vi "RT_FPGA_manualoffset_v8.vi"() -> ()   [LabVIEW 2015]
uses:
  <vilib>/rvi/interface/nirviReadWriteControl/nirviReadWriteControl.xnode
  <vilib>/rvi/interface/Simulation/niFpgaSimulationCallBeginRW.vi
  <vilib>/rvi/errors/niLvFpgaAdjustHostInterfaceError.vi
  <vilib>/rvi/interface/nirviOpenFPGA/nirviOpenFPGA.xnode
  NiFpgaLv.dll
  <vilib>/Utility/error.llb/Error Cluster From Error Code.vi
  FPGA_MPU_rev1.vi
panel:
  in  "delay in while loop execution (ms)":u32=10
  out "Acceleration (g)":cluster{dbl, dbl, dbl}(graph)
  out "Compass (deg)":cluster{dbl, dbl, dbl}(graph)
  out "Gyroscope(deg/s)":cluster{"x":dbl, "y":dbl, "z":dbl}(graph)
  in  "?":bool
  in  "stop data collection":bool
  in  "ZgyroOffH":dbl=5888.0 min=5888.0 max=6143.0
  in  "XgyroOffH":dbl=5119.0 min=4864.0 max=5119.0
  in  "YgyroOffH":dbl=5631.0 min=5376.0 max=5631.0
  in  "delay in while loop execution (ms)":u32=500
  in  "ZgyroOffL":dbl=6399.0 min=6144.0 max=6399.0
  in  "XgyroOffL":dbl=5350.0 min=5120.0 max=5375.0
  in  "YgyroOffL":dbl=5855.0 min=5632.0 max=5887.0
  in  "stop":bool
  in  "ZAccOffH":dbl=32034.0 min=32000.0 max=32255.0
  in  "XAccOffH":dbl=30483.0 min=30464.0 max=30719.0
  out "Array":u16[](array[numeric])=[5119, 5262, 5630, 5823, 5888, 6198, 6419, 6658, 6912, 7176, 7430, 7680, 7936, 8960, 14337, 14849, 27393, 30464, 30720, 31436, 31692, 32000, 32256, 27168, 26371, 6419, 6658, 14337, 14849, 9280, 9612, 9730, 10120, 10252, 10506, 10881, 25601, 27648]
  out "output array":u16[](array[numeric])
  in  "YAccOffH":dbl=31467.0 min=31232.0 max=31487.0
  out "Acceleration (g)":cluster{dbl, dbl, dbl}(graph)
  out "Gyroscope (deg/s)":cluster{dbl, dbl, dbl}(graph)
  out "Compass (deg)":cluster{dbl, dbl, dbl}(graph)
  out "array":u32[](array[numeric])
  # "Data collection"
  # "Offset"
  # "Offset control"
  # "30464 to 30719"
  # "31232 to 31487"
  # "32000 to 32255"
  # "Coarse"
  # "4864 to 5119"
  # "5376 to 5631"
  # "5888 to 6143"
  # "Fine"
  # "5120 to 5375"
  # "5632 to 5897"
  # "6144 to 6399"
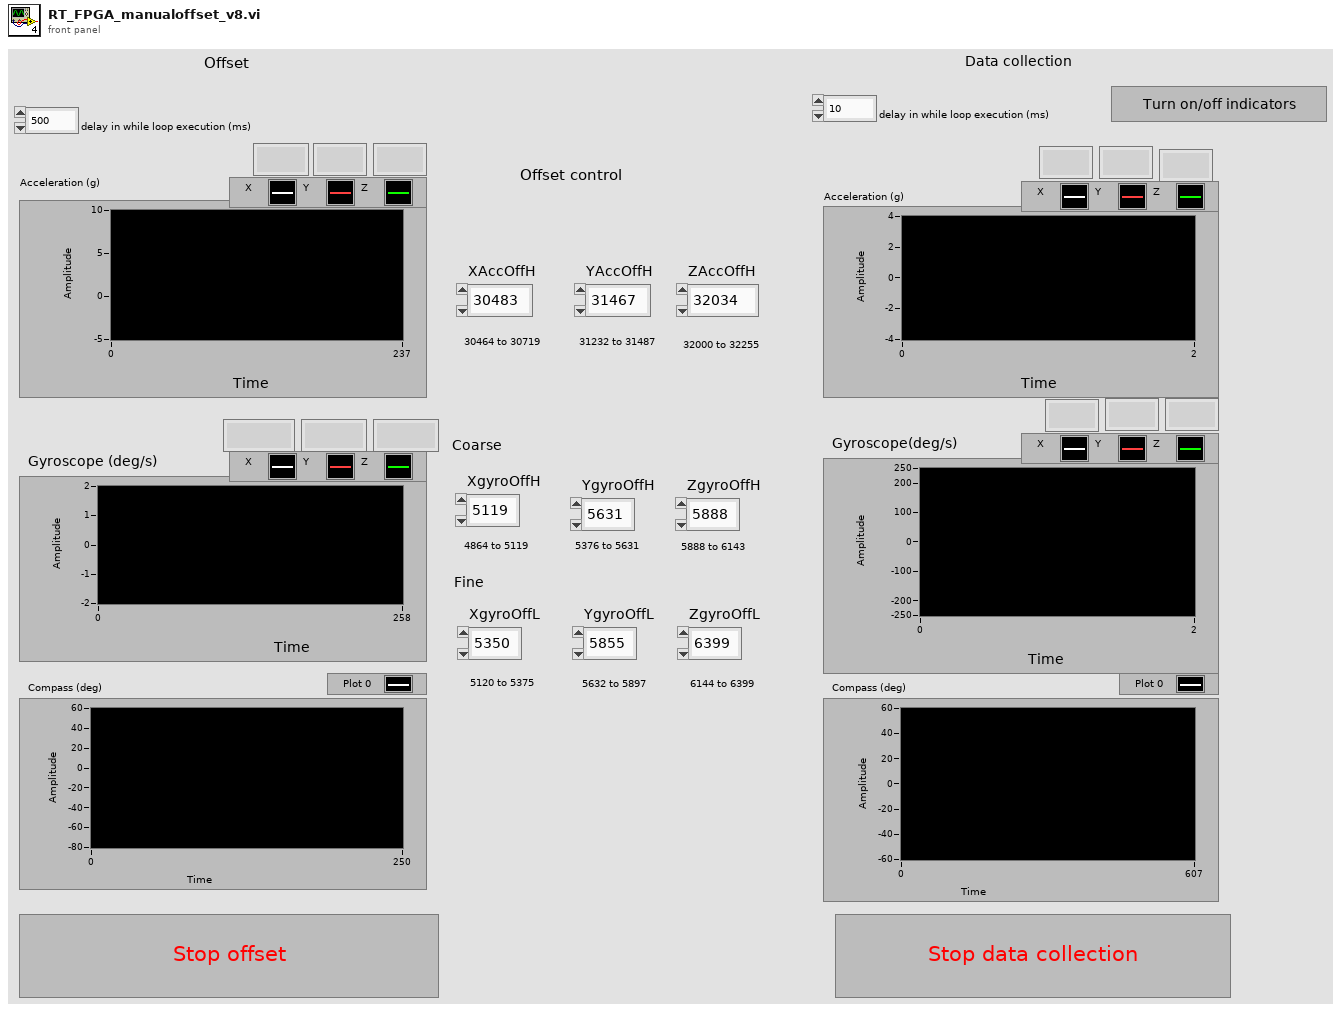
[diagram p1: front panel]
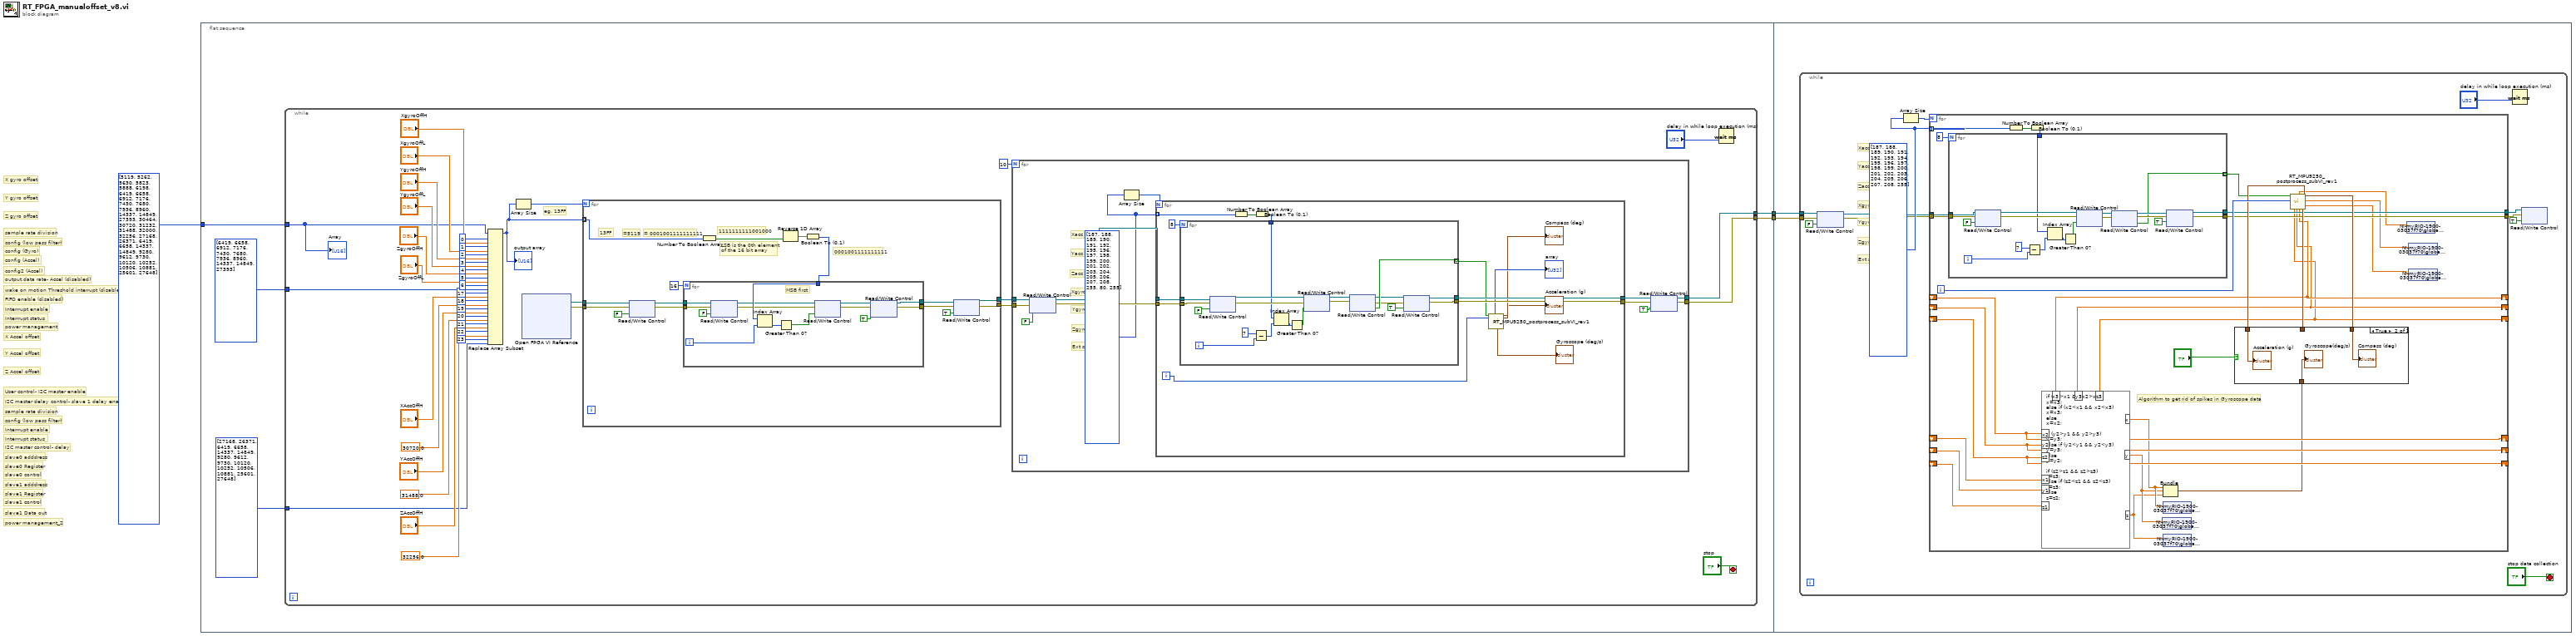
[diagram p0: block diagram]
diagram:
  # "power management_2"
  # "slave1 Data out"
  # "slave1 control"
  # "slave1 Register"
  # "slave1 adddress"
  # "slave0 control"
  # "slave0 Register"
  # "slave0 adddress"
  # "I2C master control- delay"
  # "Interrrupt status"
  # "Interrrupt enable"
  # "config (low pass filter)"
  # "sample rate division"
  # "I2C master delay control- slave 1 delay enable"
  # "User control- I2C master enable"
  # "Z Accel offset"
  # "Y Accel offset"
  # "X Accel offset"
  # "power management"
  # "Interrrupt status"
  # "Interrrupt enable"
  # "FIFO enable (disabled)"
  # "wake on motion Threshold interrupt (disabled)"
  # "output data rate- Accel (disabled)"
  # "config2 (Accel)"
  # "config (Accel)"
  # "config (Gyro)"
  # "config (low pass filter)"
  # "sample rate division"
  # "Z gyro offset"
  # "Z gyro offset"
  # "Y gyro offset"
  # "X gyro offset"
  n1 = flat-sequence {
    tunnel: u16[] [5119, 5262, 5630, 5823, 5888, 6198, 6419, 6658, 6912, 7176, 7430, 7680, 7936, 8960, 14337, 14849, 27393, 30464, 30720, 31232, 31488, 32000, 32256, 27168, 26371, 6419, 6658, 14337, 14849, 9280, 9612, 9730, 10120, 10252, 10506, 10881, 25601, 27648] -> [w8]
    tunnel: [w7] -> w2
    tunnel: [w6] -> w1
    tunnel: w2 -> [w124]
    tunnel: w1 -> [w123]
    frame #0 {
      n2 = while {
        tunnel: w8 -> [w15]
        tunnel: [w14] -> w7
        tunnel: [w13] -> w6
        tunnel: u16[] [27168, 26371, 6419, 6658, 14337, 14849, 9280, 9612, 9730, 10120, 10252, 10506, 10881, 25601, 27648] -> [w12]
        tunnel: u16[] [6419, 6658, 6912, 7176, 7430, 7680, 7936, 8960, 14337, 14849, 27393] -> [w11]
        stop <- "stop" stop-if-true
        # "eg. 13FF"
        n3 = Replace Array Subset(array=w15, new element #1="XgyroOffH", index #1=0 ("index"), new element #2="XgyroOffL", index #2=1 ("index"), new element #3="YgyroOffH", index #3=2 ("index"), new element #4="YgyroOffL", index #4=3 ("index"), new element #5="ZgyroOffH", index #5=4 ("index"), new element #6="ZgyroOffL", index #6=5 ("index"), new element #7=w11, index #7=6 ("index"), new element #8="XAccOffH", index #8=17 ("index"), new element #9=30720.0 ("XAccOffL"), index #9=18 ("index"), new element #10="YAccOffH", index #10=19 ("index"), new element #11=31488.0 ("YAccOffL"), index #11=20 ("index"), new element #12="ZAccOffH", index #12=21 ("index"), new element #13=32256.0 ("ZAccOffL"), index #13=22 ("index"), new element #14=w12, index #14=23 ("index")) -> (w17:u16[])
        "output array" <- w17
        n4 = Array Size(array=w17) -> (size(s)=w46:i32)
        n5 = xnode "Open FPGA VI Reference"() -> ("FPGA VI Reference Out"=w10:refnum<k20>, "error out"=w9:errorcluster)  [unwired: 2 in]
        n6 = for {
          N: w46 -> [_]
          tunnel: w17 -> [w108] mode=indexing
          tunnel: [w106] -> w48
          tunnel: [w105] -> w47
          tunnel: w10 -> [w104]
          tunnel: w9 -> [w103]
          # "13FF"
          # "0001001111111111"
          # "1111111111001000"
          # "= 0001001111111111"
          # "LSB is the 0th element\nof the 16 bit array"
          # "=5119"
          n7 = xnode "Read/Write Control"("FPGA VI Reference In"=w104, "error in"=w103, "CS"=FALSE ("B/DIO1 (Pin 13)")) -> ("FPGA VI Reference Out"=w96:refnum<k20>, "error out"=w95:errorcluster)
          n8 = Number To Boolean Array(number=w108) -> (Boolean array=w102:bool[])
          n9 = Reverse 1D Array(array=w102) -> (reversed array=w101:bool[])
          n10 = Boolean To (0,1)(Boolean=w101) -> (0, 1=w107:i16[])
          n11 = for {
            N: 16 -> [_]
            tunnel: w107 -> [w121]
            tunnel: [w111] -> w99
            tunnel: w96 -> [w109]
            tunnel: [w110] -> w98
            tunnel: w95 -> [w120]
            i -> [w122]
            # "MSB first"
            n12 = xnode "Read/Write Control"("FPGA VI Reference In"=w109, "error in"=w120, "SCL"=FALSE) -> ("FPGA VI Reference Out"=w115:refnum<k20>, "error out"=w114:errorcluster)
            n13 = Index Array(array=w121, index=w122) -> (element=w118:i16)
            n14 = Greater Than 0?(x=w118) -> (x > 0?=w117:bool)
            n15 = xnode "Read/Write Control"("FPGA VI Reference In"=w115, "error in"=w114, "MOSI"=w117) -> ("FPGA VI Reference Out"=w113:refnum<k20>, "error out"=w112:errorcluster)
            n16 = xnode "Read/Write Control"("FPGA VI Reference In"=w113, "error in"=w112, "SCL"=TRUE ("A/DIO0 (Pin 11)")) -> ("FPGA VI Reference Out"=w111:refnum<k20>, "error out"=w110:errorcluster)
          }
          n17 = xnode "Read/Write Control"("FPGA VI Reference In"=w99, "error in"=w98, "CS"=TRUE) -> ("FPGA VI Reference Out"=w106:refnum<k20>, "error out"=w105:errorcluster)
        }
        n18 = for {
          N: 10 -> [_]
          tunnel: w48 -> [w60]
          tunnel: w47 -> [w59]
          tunnel: [w51] -> w14
          tunnel: [w50] -> w13
          w49 = u16[] [187, 188, 189, 190, 191, 192, 195, 196, 197, 198, 199, 200, 201, 202, 203, 204, 205, 206, 207, 208, 255, 80, 255] ("Frames to Write")
          # "7"
          # "6"
          # "5"
          # "4"
          # "3"
          # "2"
          # "1"
          # "Ext sens 0"
          # "Zgyro"
          # "Ygyro"
          # "Xgyro"
          # "Zacc"
          # "Yacc"
          # "Xacc"
          n19 = xnode "Read/Write Control"("FPGA VI Reference In"=w60, "error in"=w59, "CS"=FALSE) -> ("FPGA VI Reference Out"=w58:refnum<k20>, "error out"=w57:errorcluster)
          n20 = Array Size(array=w49) -> (size(s)=w56:i32)
          n21 = for {
            N: w56 -> [_]
            tunnel: w58 -> [w71]
            tunnel: w57 -> [w70]
            tunnel: [w69] -> w53
            tunnel: [w68] -> w52
            tunnel: w49 -> [w67] mode=indexing
            i -> [w65]
            n22 = Number To Boolean Array(number=w67) -> (Boolean array=w74:bool[])
            n23 = Boolean To (0,1)(Boolean=w74) -> (0, 1=w72:i16[])
            n24 = for {
              N: 8 -> [_]
              tunnel: [w92] -> w66 mode=indexing
              tunnel: w72 -> [w80]
              tunnel: w71 -> [w79]
              tunnel: w70 -> [w78]
              tunnel: [w77] -> w69
              tunnel: [w76] -> w68
              i -> [w93]
              n25 = xnode "Read/Write Control"("FPGA VI Reference In"=w79, "error in"=w78, "SCL"=FALSE ("B/DIO5 (Pin 21)")) -> ("FPGA VI Reference Out"=w85:refnum<k20>, "error out"=w86:errorcluster)
              n26 = Subtract(x=7, y=w93) -> (x-y=w88:i32)
              n27 = Index Array(array=w80, index=w88) -> (element=w75:i16)
              n28 = Greater Than 0?(x=w75) -> (x > 0?=w90:bool)
              n29 = xnode "Read/Write Control"("FPGA VI Reference In"=w85, "error in"=w86, "MOSI"=w90) -> ("FPGA VI Reference Out"=w84:refnum<k20>, "error out"=w83:errorcluster)
              n30 = xnode "Read/Write Control"("FPGA VI Reference In"=w84, "error in"=w83) -> ("FPGA VI Reference Out"=w82:refnum<k20>, "error out"=w81:errorcluster, "MISO"=w92:bool)
              n31 = xnode "Read/Write Control"("FPGA VI Reference In"=w82, "error in"=w81, "SCL"=TRUE ("A/DIO0 (Pin 11)")) -> ("FPGA VI Reference Out"=w77:refnum<k20>, "error out"=w76:errorcluster)
            }
            n32 = call "RT_MPU9250_postprocess_subVI_rev1.vi"("readings in bits"=w66, "number of samples"=w65) -> ("readings in decimal"=→"array":u32[], "Gyroscope (deg/s)"=→"Gyroscope (deg/s)":cluster{dbl, dbl, dbl}, "Acceleration (g)"=→"Acceleration (g)":cluster{dbl, dbl, dbl}, "Compass"=→"Compass (deg)":cluster{dbl, dbl, dbl})  [unwired: 5 in, 9 out]
          }
          n33 = xnode "Read/Write Control"("FPGA VI Reference In"=w53, "error in"=w52, "CS"=TRUE ("B/DIO1 (Pin 13)")) -> ("FPGA VI Reference Out"=w51:refnum<k20>, "error out"=w50:errorcluster)
        }
        n34 = Wait (ms)(milliseconds to wait="delay in while loop execution (ms)") -> ()  [unwired: 1 out]
        "Array" <- w15
      }
    }
    frame #1 {
      n35 = while {
        tunnel: w124 -> [w133]
        tunnel: w123 -> [w132]
        stop <- "stop data collection" stop-if-true
        w135 = u16[] [187, 188, 189, 190, 191, 192, 193, 194, 195, 196, 197, 198, 199, 200, 201, 202, 203, 204, 205, 206, 207, 208, 255] ("Frames to Write")
        # "7"
        # "6"
        # "5"
        # "4"
        # "3"
        # "2"
        # "1"
        # "Ext sens 0"
        # "Zgyro"
        # "Ygyro"
        # "Xgyro"
        # "Zacc"
        # "Yacc"
        # "Xacc"
        n36 = xnode "Read/Write Control"("FPGA VI Reference In"=w133, "error in"=w132, "CS"=FALSE) -> ("FPGA VI Reference Out"=w131:refnum<k20>, "error out"=w130:errorcluster)
        n37 = Array Size(array=w135) -> (size(s)=w136:i32)
        n38 = for {
          N: w136 -> [_]
          tunnel: w135 -> [w164] mode=indexing
          tunnel: w131 -> [w156]
          tunnel: w130 -> [w155]
          tunnel: [w154] -> w128
          tunnel: [w153] -> w127
          shift-right: [w152] -> _
          shift-left: _ -> [w147]
          shift-right: [w147] -> _
          shift-left: _ -> [w151]
          shift-right: [w150] -> _
          shift-left: _ -> [w149]
          shift-right: [w149] -> _
          shift-left: _ -> [w148]
          shift-right: [w146] -> _
          shift-left: _ -> [w145]
          shift-right: [w145] -> _
          shift-left: _ -> [w144]
          i -> [w162]
          # "Algorithm to get rid of spikes in Gyroscope data"
          n39 = Number To Boolean Array(number=w164) -> (Boolean array=w166:bool[])
          n40 = Boolean To (0,1)(Boolean=w166) -> (0, 1=w163:i16[])
          n41 = for {
            N: 8 -> [_]
            tunnel: [w172] -> w158 mode=indexing
            tunnel: w163 -> [w173]
            tunnel: w156 -> [w176]
            tunnel: w155 -> [w175]
            tunnel: [w171] -> w154
            tunnel: [w170] -> w153
            i -> [w174]
            n42 = xnode "Read/Write Control"("FPGA VI Reference In"=w176, "error in"=w175, "SCL"=FALSE) -> ("FPGA VI Reference Out"=w183:refnum<k20>, "error out"=w182:errorcluster)
            n43 = Subtract(x=7, y=w174) -> (x-y=w187:i32)
            n44 = Index Array(array=w173, index=w187) -> (element=w186:i16)
            n45 = Greater Than 0?(x=w186) -> (x > 0?=w184:bool)
            n46 = xnode "Read/Write Control"("FPGA VI Reference In"=w183, "error in"=w182, "MOSI"=w184) -> ("FPGA VI Reference Out"=w181:refnum<k20>, "error out"=w180:errorcluster)
            n47 = xnode "Read/Write Control"("FPGA VI Reference In"=w181, "error in"=w180) -> ("FPGA VI Reference Out"=w178:refnum<k20>, "error out"=w177:errorcluster, "MISO"=w172:bool)
            n48 = xnode "Read/Write Control"("FPGA VI Reference In"=w178, "error in"=w177, "SCL"=TRUE) -> ("FPGA VI Reference Out"=w171:refnum<k20>, "error out"=w170:errorcluster)
          }
          n49 = call "RT_MPU9250_postprocess_subVI_rev1.vi"("readings in bits"=w158, "number of samples"=w162) -> ("Zgyro"=w146:dbl, "Ygyro"=w150:dbl, "XAccel"=w140:dbl, "Gyroscope (deg/s)"=w159:cluster{dbl, dbl, dbl}, "Xgyro"=w152:dbl, "Acceleration (g)"=w160:cluster{dbl, dbl, dbl}, "Compass"=w161:cluster{dbl, dbl, dbl}, "YAccel"=w141:dbl, "ZAccel"=w142:dbl)  [unwired: 5 in, 4 out]
          n50 = formula code="if (x2>x1 && x2>x3)\nx=x3;\nelse if (x2<x1 && x2<x3)\nx=x3;\nelse\nx=x2;\n\nif (y2>y1 && y2>y3)\ny=y3;\nelse if (y2<y1 && y2<y3)\ny=y3;\nelse\ny=y2;\n\nif (z2>z1 && z2>z3)\nz=z3;\nelse if (z2<z1 && z2<z3)\nz=z3;\nelse\nz=z2;"("x1"=w151, "x3"=w152, "x2"=w147, "y3"=w150, "y2"=w149, "y1"=w148, "z3"=w146, "z1"=w144, "z2"=w145) -> ("x"=w139:dbl, "y"=w138:dbl, "z"=w137:dbl)
          n51 = shared-variable "NI-myRIO-1900-03037f70\\global variable library.lvlib\\YG"(w138) -> ()  [unwired: 1 in, 1 out]
          n52 = shared-variable "NI-myRIO-1900-03037f70\\global variable library.lvlib\\XG"(w139) -> ()  [unwired: 1 in, 1 out]
          n53 = shared-variable "NI-myRIO-1900-03037f70\\global variable library.lvlib\\ZG"(w137) -> ()  [unwired: 1 in, 1 out]
          n54 = Bundle("x"=w139, "y"=w138, "z"=w137) -> (w143:cluster{"x":dbl, "y":dbl, "z":dbl})  [unwired: 1 in]
          n55 = case shown="True" "?" {
            tunnel: w161 -> [_ w169]
            tunnel: w160 -> [_ w168]
            tunnel: w159 -> [_ _]
            tunnel: w143 -> [_ w167]
            frame False {
            }
            frame True {
              "Acceleration (g)" <- w168
              "Compass (deg)" <- w169
              "Gyroscope(deg/s)" <- w167
            }
          }
          n56 = shared-variable "NI-myRIO-1900-03037f70\\global variable library.lvlib\\XA"(w140) -> ()  [unwired: 1 in, 1 out]
          n57 = shared-variable "NI-myRIO-1900-03037f70\\global variable library.lvlib\\YA"(w141) -> ()  [unwired: 1 in, 1 out]
          n58 = shared-variable "NI-myRIO-1900-03037f70\\global variable library.lvlib\\ZA"(w142) -> ()  [unwired: 1 in, 1 out]
        }
        n59 = Wait (ms)(milliseconds to wait="delay in while loop execution (ms)") -> ()  [unwired: 1 out]
        n60 = xnode "Read/Write Control"("FPGA VI Reference In"=w128, "error in"=w127, "CS"=TRUE) -> ()  [unwired: 2 out]
      }
    }
  }
